vi "Handle Messages.vi"(8 "error in (no error)":errorcluster, 9 "Message Data":variant, 10 "Message":string, 11 "Process In":refnum<class>) -> (0 "error out":errorcluster, 3 "Process Out":refnum<class>)   [LabVIEW 2020]
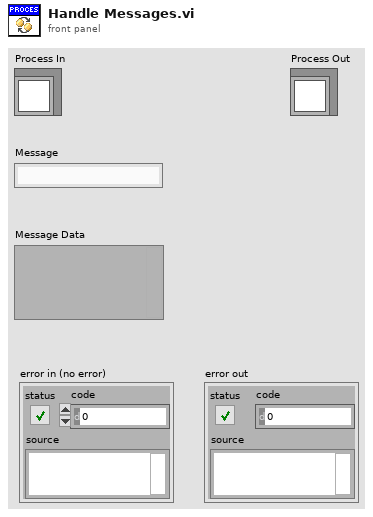
[diagram p1: front panel]
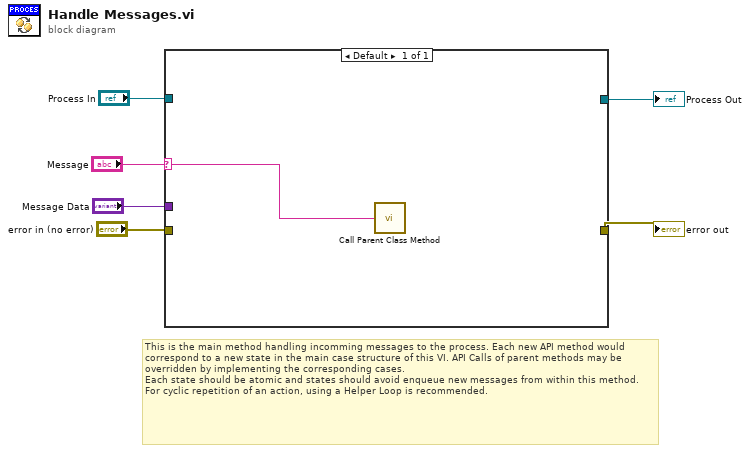
[diagram p0: block diagram]
diagram:
  # "This is the main method handling incomming messages to the process. Each new API method would correspond to a new state in the main case structure of this VI. API Calls of parent methods may be overridden by implementing the corresponding cases.\nEach state should be atomic and states should avoid enqueue new messages from within this method. For cyclic repetition of an action, using a Helper Loop is recommended."
  n1 = case shown="Default" "Message" {
    selector: "Message" -> [w11]
    tunnel: [w8] -> w5
    tunnel: "error in (no error)" -> [w7]
    tunnel: [w10] -> w3
    tunnel: "Process In" -> [w9]
    tunnel: "Message Data" -> [_]
    frame Default {
      n2 = call-parent "Call Parent Class Method"(w11) -> ()
    }
  }
  "error out" <- w5
  "Process Out" <- w3
